vi "test.vi"() -> ()   [LabVIEW 2020]
uses:
  x64/Release/Passing.dll
panel:
  in  "size":i32=8
  out "arr 2":dbl[](array[numeric])=[0.5, 1.5, 2.5, 3.5, 4.5, 5.5]
  in  "arr in":dbl[](array[numeric])=[0.0, 1.25, 0.0, 5.0, 0.0, 8.0]
  out "arr":dbl[](array[numeric])=[0.5, 1.5, 2.5, 3.5, 4.5, 5.5]
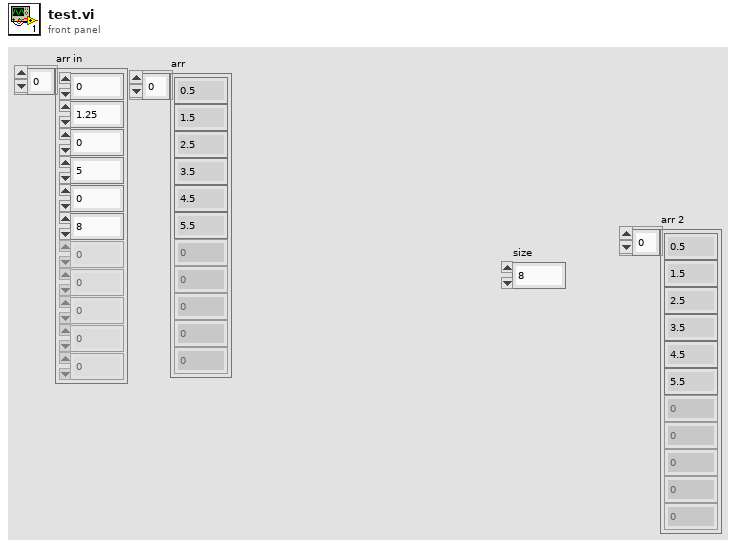
[diagram p1: front panel]
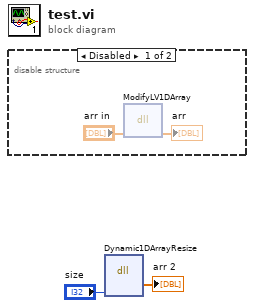
[diagram p0: block diagram]
diagram:
  n1 = disable-structure shown="Disabled" {
    frame Disabled {
      n2 = dll-call lib="E:/Practice/Lv/dll/CppDllForLv/x64/Release/Passing.dll" fn="ModifyLV1DArray"("arr"="arr in") -> ("arr"=→"arr":dbl[])  [unwired: 4 in, 2 out]
    }
    frame Enabled {
    }
  }
  n3 = dll-call lib="E:/Practice/Lv/dll/CppDllForLv/x64/Release/Passing.dll" fn="Dynamic1DArrayResize"("size"="size") -> ("arr"=→"arr 2":dbl[])  [unwired: 6 in, 2 out]
